vi "test Minor Frame Address Pairs In Log.vi"(8 "error in (no error)":errorcluster, 11 "TestCase in":refnum<class "Logging Loopback.lvclass">) -> (0 "error out":errorcluster, 3 "TestCase out":refnum<class "Logging Loopback.lvclass">)   [LabVIEW 2020, in "Logging Loopback.lvclass"]
uses:
  Logging Loopback.lvclass
  Logging Loopback.lvclass/Logging Loopback.ctl
  6070ecc1-7a7f-4aba-84f3-8f274e3c644e.vi
  <vilib>/WebDAVClient/Advanced/Get Buffer.vi
  <vilib>/addons/_JKI Toolkits/VI Tester/TestCase.llb/TestCase.lvclass
  <vilib>/WebDAVClient/NI_WebDAV.lvlib
  C:/dev/git/niveristand-custom-device-testing-tools/VeriStandTestCase/VeriStandTestCase.lvclass
  C:/Program Files (x86)/National Instruments/LabVIEW 2020/vi.lib/addons/_JKI Toolkits/VI Tester/TestCase.llb/TestCase.lvclass
  C:/dev/git/niveristand-aim-milStd1553-custom-device/Source/Custom Device Support/Tests/System/Logging Loopback/Logging Loopback.lvclass
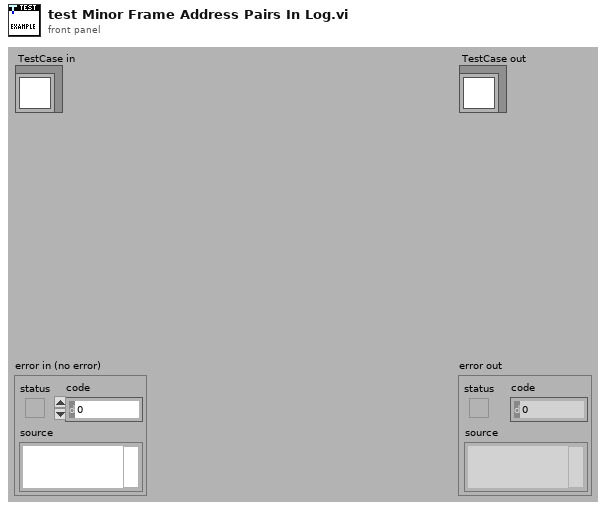
[diagram p1: front panel]
types:
  T1 = typedef "NI_WebDAV.lvlib/SessionHandle.ctl" = refnum<k1>
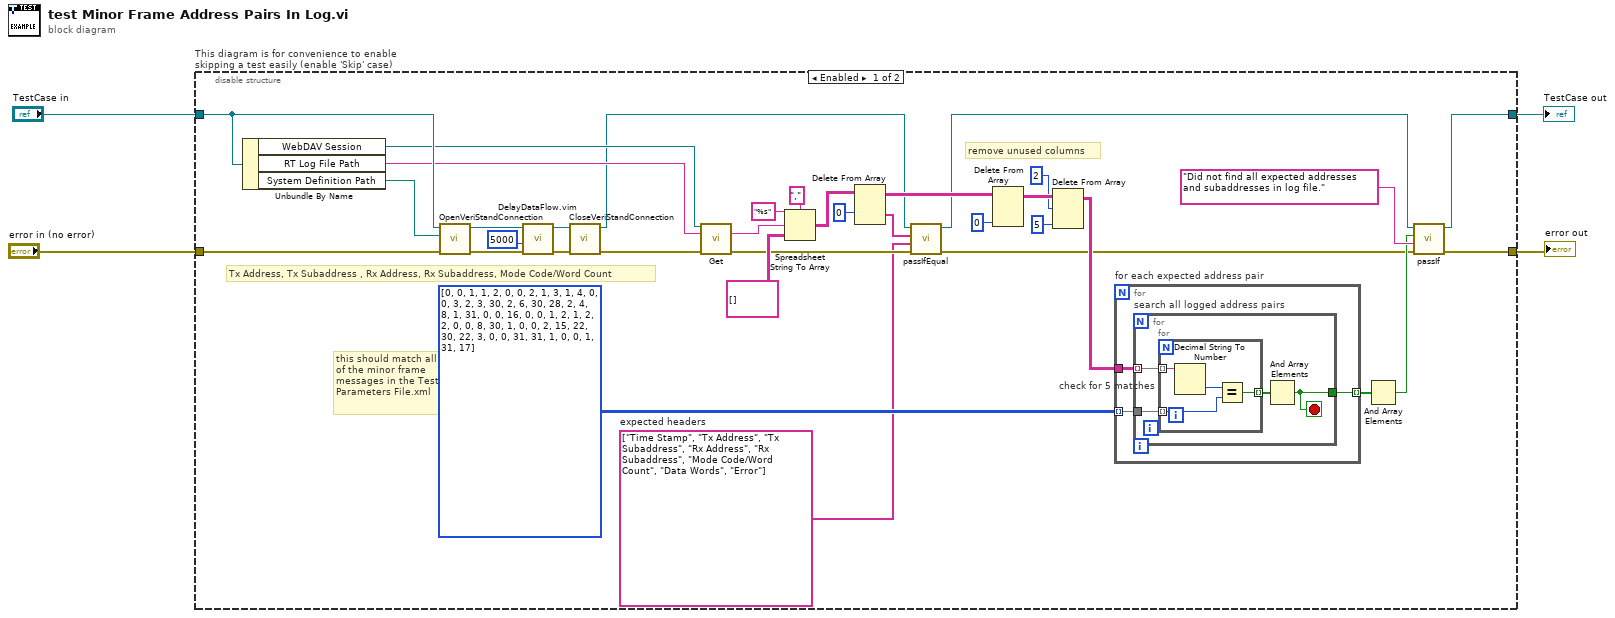
[diagram p0: block diagram]
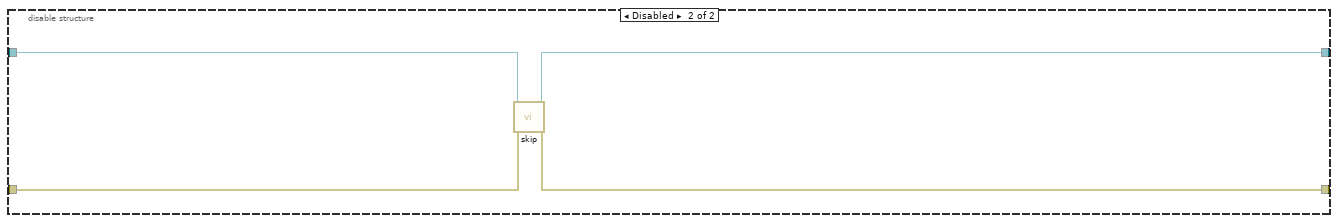
[diagram p2: hidden frame]
diagram:
  n1 = disable-structure "This diagram is for convenience to enable skipping a test easily (enable 'Skip' case)" shown="Enabled" {
    disable-tunnel: "TestCase in" -> [w35 w53]
    disable-tunnel: [w23 w51] -> w1
    disable-tunnel: [w24 w52] -> w3
    disable-tunnel: "error in (no error)" -> [w38 w50]
    frame Enabled {
      w6 = string[] ["Time Stamp", "Tx Address", "Tx Subaddress", "Rx Address", "Rx Subaddress", "Mode Code/Word Count", "Data Words", "Error"]  # expected headers
      # "remove unused columns"
      # "this should match all of the minor frame messages in the Test Parameters File.xml"
      # "Tx Address, Tx Subaddress , Rx Address, Rx Subaddress, Mode Code/Word Count"
      n2 = Unbundle By Name(w35) -> ("WebDAV Session"=w30:T1, "RT Log File Path"=w29:string, "System Definition Path"=w36:path)
      n3 = call-dynamic "OpenVeriStandConnection.vi"("error in (no error)"=w38, "System Definition File"=w36, "VeriStand Test Case in"=w35) -> ("error out"=w37:errorcluster, "VeriStand Test Case out"=w32:refnum<class "Logging Loopback.lvclass">)  [unwired: 6 in, 1 out]
      n4 = call "DelayDataFlow.vim"("value in"=w37, "milliseconds to wait"=u32 5000) -> ("value out"=w34:errorcluster)  [unwired: 2 in, 1 out]
      n5 = call-dynamic "CloseVeriStandConnection.vi"("error in (no error)"=w34, "VeriStand Test Case in"=w32) -> ("error out"=w31:errorcluster, "VeriStand Test Case out"=w9:refnum<class "Logging Loopback.lvclass">)  [unwired: 8 in]
      n6 = call-poly <vilib>:"Get.vi"("session handle"=w30, "relative uri"=w29, "error in (no error)"=w31) -> ("data"=w28:string, "error out"=w11:errorcluster)  [unwired: 10 in, 1 out]
      n7 = Spreadsheet String To Array(delimiter (Tab)=",", format string="%s", spreadsheet string=w28, array type (2D Dbl)=string[][] []) -> (array=w13:string[][])
      n8 = Delete From Array(array=w13, index (row)=0) -> (deleted portion=w7:string[], array with subset deleted=w12:string[][])  [unwired: 2 in]
      n9 = call-dynamic "passIfEqual.vi"("error in (no error)"=w11, "y"=w6, "x"=w7, "TestCase in"=w9) -> ("error out"=w10:errorcluster, "TestCase out"=w8:refnum<class "Logging Loopback.lvclass">)  [unwired: 6 in]
      n10 = Delete From Array(array=w12, index (col)=0 ("disabled index (col)")) -> (array with subset deleted=w19:string[][])  [unwired: 2 in, 1 out]
      n11 = Delete From Array(array=w19, length=2, index (col)=5 ("disabled index (col)")) -> (array with subset deleted=w17:string[][])  [unwired: 1 in, 1 out]
      n12 = for "for each expected address pair" {
        tunnel: w17 -> [w41]
        tunnel: i32[][] [[0, 0, 1, 1, 2], [0, 0, 2, 1, 3], [1, 4, 0, 0, 3], [2, 3, 30, 2, 6], [30, 28, 2, 4, 8], [1, 31, 0, 0, 16], [0, 0, 1, 2, 1], [2, 2, 0, 0, 8], [30, 1, 0, 0, 2], [15, 22, 30, 22, 3], [0, 0, 31, 31, 1], [0, 0, 1, 31, 17]] -> [w40] mode=indexing
        tunnel: [w39] -> w15 mode=indexing
        n13 = for "search all logged address pairs" {
          tunnel: w41 -> [w45] mode=indexing
          tunnel: w40 -> [w44]
          tunnel: [w42] -> w39
          stop <- w42 stop-if-true
          n14 = for "check for 5 matches" {
            tunnel: w45 -> [w49] mode=indexing
            tunnel: w44 -> [w47] mode=indexing
            tunnel: [w46] -> w43 mode=indexing
            n15 = Decimal String To Number(string=w49) -> (number=w48:i32)  [unwired: 2 in, 1 out]
            n16 = Equal?(x=w48, y=w47) -> (x = y?=w46:bool)
          }
          n17 = And Array Elements(Boolean array=w43) -> (logical AND=w42:bool)
        }
      }
      n18 = And Array Elements(Boolean array=w15) -> (logical AND=w14:bool)
      n19 = call-dynamic "passIf.vi"("error in (no error)"=w10, "message (\"\")"="Did not find all expected addresses and subaddresses in log file." ("message (\"\")"), "pass"=w14, "TestCase in"=w8) -> ("error out"=w24:errorcluster, "TestCase out"=w23:refnum<class "Logging Loopback.lvclass">)  [unwired: 6 in]
    }
    frame Disabled {
      # "skip test result while test is under development"
      n20 = call <vilib>:"skip.vi"("error in (no error)"=w50, "TestCase in"=w53) -> ("error out"=w52:errorcluster, "TestCase out"=w51:refnum<class "Logging Loopback.lvclass">)  [unwired: 8 in]
    }
  }
  "error out" <- w3
  "TestCase out" <- w1
